vi "Write Clear Time.vi"(8 "error in (no error)":errorcluster, 10 "Clear Time":timestamp, 11 "AE in":refnum<class "AE.lvclass">) -> (0 "error out":errorcluster, 3 "AE out":refnum<class "AE.lvclass">)   [LabVIEW 2014, in "CS++ProcessVariables.lvlib" / "AE.lvclass"]
doc: "Write attribute value."
uses:
  AE.lvclass
  AE.lvclass/AE.ctl
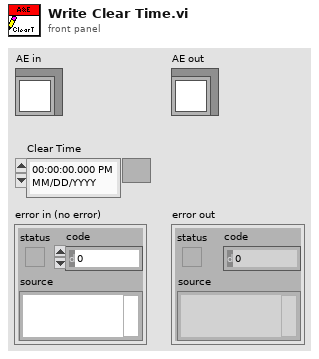
[diagram p1: front panel]
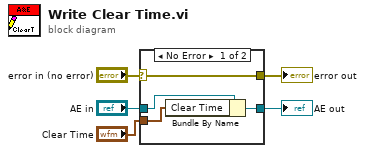
[diagram p0: block diagram]
diagram:
  n1 = case shown="No Error" "error in (no error)" {
    selector: "error in (no error)" -> [w9 w10]
    tunnel: [w9 w10] -> w4
    tunnel: [w7 w11] -> w2
    tunnel: "AE in" -> [w8 w11]
    tunnel: "Clear Time" -> [w6 _]
    frame No Error {
      n2 = Bundle By Name(cluster=w8, "Clear Time"=w6) -> (w7:refnum<class "AE.lvclass">)
    }
    frame Error {
    }
  }
  "error out" <- w4
  "AE out" <- w2
